vi "ConfigTrigger.vi"(8 "error in (no error)":errorcluster, 11 "Agilent_3458 in":refnum<class "Agilent_3458.lvclass">) -> (0 "error out":errorcluster, 3 "Agilent_3458 out":refnum<class "Agilent_3458.lvclass">)   [LabVIEW 2018, in "DigitizerPlugins.lvlib" / "Agilent_3458.lvclass"]
uses:
  Agilent_3458.lvclass
  F:/Projects/ICDAS/NistPluggableModules/Digitizer/DigitizerPlugins/DigitizerBaseClass/DigitizerBase.lvclass
  DigitizerBaseClass/DigitizerBase.lvclass/DigitizerBase.ctl
  DigitizerBaseClass/Accessors/Read Handle.vi
  DigitizerBaseClass/Accessors/Read Trigger.vi
  DigitizerBaseClass/Accessors/Read Acquisition.vi
  <instrlib>/Agilent 3458/Agilent 3458.lvlib
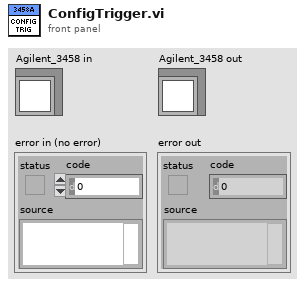
[diagram p1: front panel]
types:
  T1 = typedef "DigitizerPlugins.lvlib/DigitizerBase.lvclass/Trigger.ctl" = cluster{"Source":string, "Delay":dbl, "Holdoff":dbl, "PretriggerSamples":i32, "Sources":T2[]}
  T2 = typedef "DigitizerPlugins.lvlib/DigitizerBase.lvclass/TrigSource.ctl" = cluster{"Name":string, "Coupling":enum16{"AC", "DC", "HF Reject", "LF Reject", "Noise Reject"}, "Hysteresis":dbl, "Level":dbl, "Slope":enum16{"Positive", "Negative"}, "Type":enum16{"Edge", "Width", "Runt", "Glitch", "TV", "Window"}}
  T3 = typedef "DigitizerPlugins.lvlib/DigitizerBase.lvclass/Acquisition.ctl" = cluster{"SampleRate":dbl, "RecordSize":i32, "NumRecords":i32, "SampleMode":i32, "Timeout (ms)":i32}
  T4 = enum16{"AC", "DC", "HF Reject", "LF Reject", "Noise Reject"}
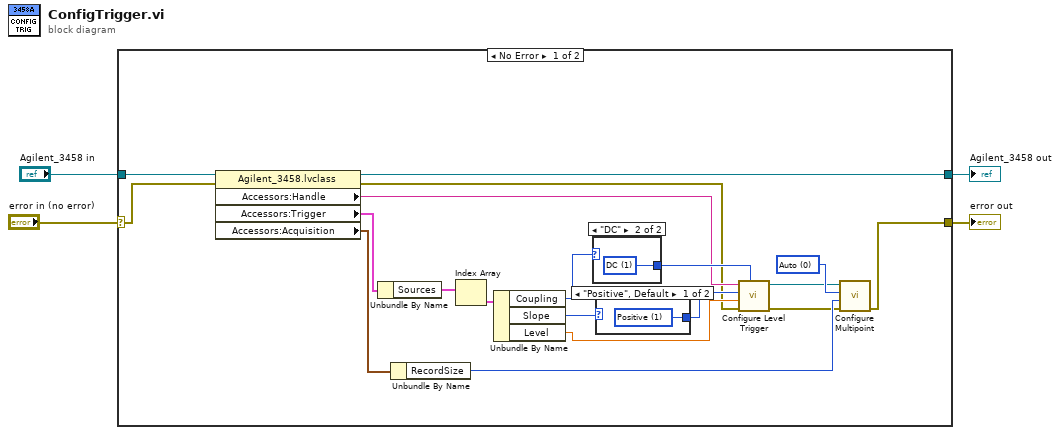
[diagram p0: block diagram]
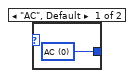
[diagram p2: hidden frame]
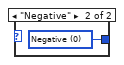
[diagram p3: hidden frame]
diagram:
  n1 = case shown="No Error" "error in (no error)" {
    selector: "error in (no error)" -> [w22 w28]
    tunnel: [w21 w29] -> w2
    tunnel: "Agilent_3458 in" -> [w23 w29]
    tunnel: [w20 w28] -> w1
    frame No Error {
      w19 = u16 0 items=["Auto", "External", "Level", "Line", "Synchronous"] ("Trigger Type (0:Auto)")
      n2 = property class="Agilent_3458.lvclass"(reference=w23, error in=w22) -> (reference out=w21:refnum<class "Agilent_3458.lvclass">, error out=w9:errorcluster, "Accessors:Handle"=w13:string, "Accessors:Trigger"=w11:T1, "Accessors:Acquisition"=w8:T3)
      n3 = Unbundle By Name(w11) -> ("Sources"=w18:T2[])
      n4 = Unbundle By Name(w8) -> ("RecordSize"=w6:i32)
      n5 = Index Array(array=w18) -> (element=w17:T2)  [unwired: 1 in]
      n6 = Unbundle By Name(w17) -> ("Coupling"=w15:T4, "Slope"=w16:enum16{"Positive", "Negative"}, "Level"=w10:dbl)
      n7 = case shown="\"DC\"" w15 {
        tunnel: [w24 w25] -> w14
        frame "AC", Default {
          w24 = u16 0 items=["AC", "DC"] ("Coupling (0:AC)")
        }
        frame "DC" {
          w25 = u16 1 items=["AC", "DC"] ("Coupling (0:AC)")
        }
      }
      n8 = case shown="\"Positive\", Default" w16 {
        tunnel: [w26 w27] -> w12
        frame "Positive", Default {
          w26 = u16 1 items=["Negative", "Positive"] ("Slope (1:Positive)")
        }
        frame "Negative" {
          w27 = u16 0 items=["Negative", "Positive"] ("Slope (1:Positive)")
        }
      }
      n9 = call <instrlib>:"Configure Level Trigger.vi"("Coupling (0:AC)"=w14, "error in (no error)"=w9, "Percentage (0%)"=w10, "Slope (1:Positive)"=w12, "VISA resource name"=w13) -> ("error out"=w5:errorcluster, "VISA resource name out"=w7:refnum<visa-resource-name>)  [unwired: 5 in]
      n10 = call <instrlib>:"Configure Multipoint.vi"("error in (no error)"=w5, "Sample Count (1)"=w6, "Trigger Type (0:Auto)"=w19, "VISA resource name"=w7) -> ("error out"=w20:errorcluster)  [unwired: 6 in, 1 out]
    }
    frame Error {
    }
  }
  "error out" <- w1
  "Agilent_3458 out" <- w2
